vi "action.vi"(0 "HB_Simple_Add":refnum<class "HB_Simple_Add.lvclass">, 2 "HGF_Visitable":refnum<class "HGF_Visitable.lvclass">, 5 "error in (no error)":errorcluster) -> (14 "dup HB_Simple_Add":refnum<class "HB_Simple_Add.lvclass">, 16 "dup HGF_Visitable":refnum<class "HGF_Visitable.lvclass">, 19 "error out":errorcluster)   [LabVIEW 2009, in "HB_BaseClass_Examples.lvlib" / "HB_Simple_Add.lvclass"]
doc: "This is a dynamic dispatch VI that is called from Visitor.visit(). It will call member VIs of Visitable to perform the requested action which means: calling public methods of Visitable child class.\n\n<B>Hint:</B> This method is abstract and need to be implemented by child classes."
uses:
  HB_Simple_Add.lvclass
  lib.lib/HGF_LVC/HGF_BaseClasses/HGF_Visitable/HGF_Visitable.lvclass
  HB_Simple.lvclass
  HB_Simple_Add.lvclass/HB_Simple_Add.ctl
  lib.lib/HGF_LVC/HGF_BaseClasses/HGF_NetworkVisitor/HGF_NetworkVisitor.lvclass
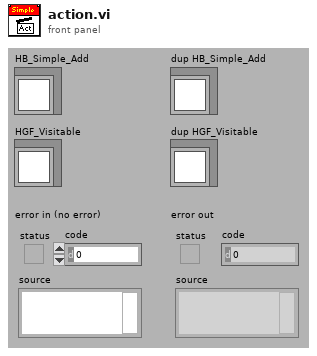
[diagram p1: front panel]
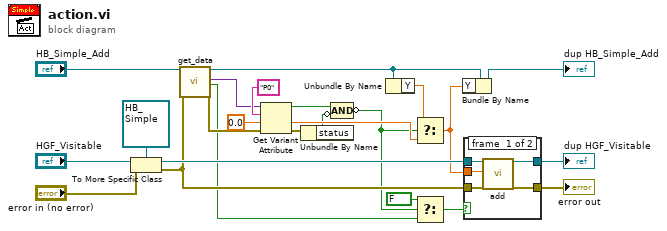
[diagram p0: block diagram]
diagram:
  n1 = To More Specific Class(target class=refnum<class "HB_Simple.lvclass"> refnum ("HB_HGF_Test.lvlib:HB_Simple.lvclass"), reference="HGF_Visitable", error in="error in (no error)") -> (specific class reference=w20:refnum<class "HB_Simple.lvclass">, error out=w12:errorcluster)
  n2 = call "get_data.vi"("HGF_NetworkData"="HB_Simple_Add", "error in (no error)"=w12) -> ("dup HGF_NetworkData"=w7:refnum<class "HB_Simple_Add.lvclass">, "data"=w11:variant, "no link"=w9:bool, "error out"=w10:errorcluster)  [unwired: 14 out]
  n3 = Get Variant Attribute(Variant=w11, name="P0", default value (empty Variant)=0.0, error in=w10) -> (found=w2:bool, value=w14:dbl, error out=w3:errorcluster)  [unwired: 1 out]
  n4 = Unbundle By Name(w3) -> ("status"=w4:bool)
  n5 = Compound Arithmetic op=AND(w2, invert w4) -> (invert w1:bool)
  n6 = Unbundle By Name(w7) -> ("Y"=w8:dbl)
  n7 = Select(t=w8, s=w1, f=w14) -> (s? t:f=w5:dbl)
  n8 = Select(t=FALSE, s=w1, f=w9) -> (s? t:f=w17:bool)
  n9 = Bundle By Name(cluster=w7, "Y"=w5) -> (→"dup HB_Simple_Add":refnum<class "HB_Simple_Add.lvclass">)
  n10 = case shown="False" w17 {
    tunnel: [w29 w31] -> w22
    tunnel: [w28 w30] -> w21
    tunnel: w20 -> [w27 w31]
    tunnel: w5 -> [w26 _]
    tunnel: w12 -> [w25 w30]
    frame #0 {
      n11 = call "add.vi"("HB_Simple in"=w27, "y"=w26, "error in (no error)"=w25) -> ("HB_Simple out"=w29:refnum<class "HB_Simple.lvclass">, "error out"=w28:errorcluster)  [unwired: 15 out]
    }
    frame #1 {
    }
  }
  "error out" <- w21
  "dup HGF_Visitable" <- w22
